vi "Jenkins - Call Build.vi"(8 "error in (no error)":errorcluster, 9 "Parameters":variant, 10 "Script Job Name (Within Build Script Folder)":string, 11 "IP Address":string) -> (0 "error out":errorcluster)   [LabVIEW 2014]
uses:
  <vilib>/httpClient/LabVIEWHTTPClient.lvlib
  <vilib>/wsapi/NI_WebServices.lvlib
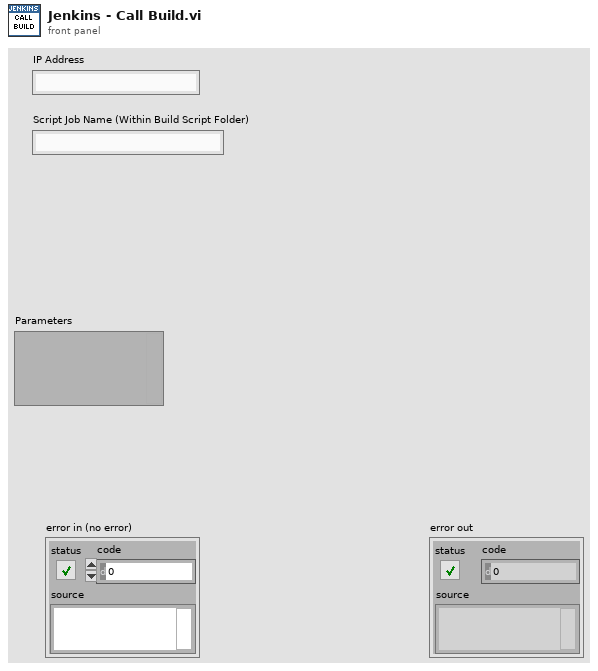
[diagram p1: front panel]
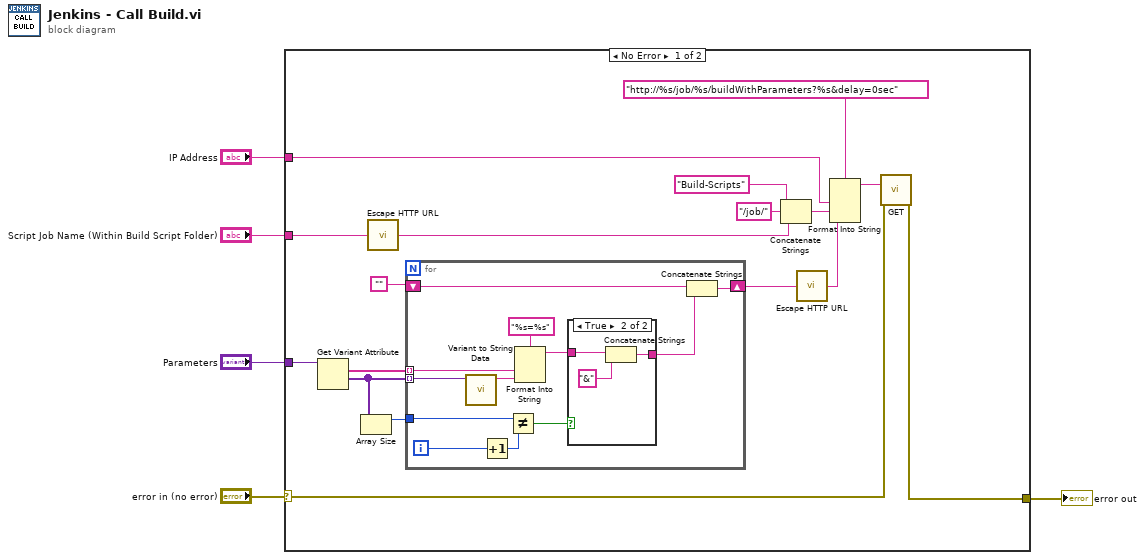
[diagram p0: block diagram]
diagram:
  n1 = case shown="No Error" "error in (no error)" {
    selector: "error in (no error)" -> [w11 w39]
    tunnel: "Script Job Name (Within Build Script Folder)" -> [w10 _]
    tunnel: "IP Address" -> [w18 _]
    tunnel: [w17 w39] -> w3
    tunnel: "Parameters" -> [w8 _]
    frame No Error {
      n2 = Get Variant Attribute(Variant=w8) -> (names=w7:string[], values=w6:variant[])  [unwired: 3 in, 2 out]
      n3 = Array Size(array=w6) -> (size(s)=w15:i32)
      n4 = call <vilib>:"Escape HTTP URL.vi"("unescaped string in"=w10) -> ("escaped string out"=w9:string)
      n5 = for {
        shift-right: [w32] -> w14
        shift-left: "" -> [w33]
        tunnel: w15 -> [w29]
        tunnel: w7 -> [w25] mode=indexing
        tunnel: w6 -> [w24] mode=indexing
        i -> [w31]
        n6 = call "Variant to String Data.vi"("Variant"=w24) -> ("String Data"=w23:string)  [unwired: 9 in, 1 out]
        n7 = Increment(x=w31) -> (x+1=w30:i32)
        n8 = Not Equal?(x=w29, y=w30) -> (x != y?=w28:bool)
        n9 = Format Into String(format string="%s=%s", w25, w23) -> (resulting string=w27:string)  [unwired: 2 in, 1 out]
        n10 = case shown="True" w28 {
          tunnel: w27 -> [w35 w38]
          tunnel: [w35 w36] -> w26
          frame False {
          }
          frame True {
            n11 = Concatenate Strings(w38, "&" ("string")) -> (w36:string)
          }
        }
        n12 = Concatenate Strings(w33, w26) -> (w32:string)
      }
      n13 = Concatenate Strings("Build-Scripts" ("JSON"), "/job/" ("string"), w9) -> (w19:string)
      n14 = call <vilib>:"Escape HTTP URL.vi"("unescaped string in"=w14) -> ("escaped string out"=w13:string)
      n15 = Format Into String(format string="http://%s/job/%s/buildWithParameters?%s&delay=0sec", w18, w19, w13) -> (resulting string=w22:string)  [unwired: 2 in, 1 out]
      n16 = call <vilib>:"GET.vi"("url"=w22, "error in (no error)"=w11) -> ("error out"=w17:errorcluster)  [unwired: 10 in, 3 out]
    }
    frame Error {
    }
  }
  "error out" <- w3
